vi "Parse Data DualHeading(SubVI).vi"(11 "Parse Data Array":string[](array[string])) -> (3 "Heading":dbl)   [LabVIEW 2019]
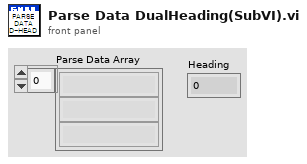
[diagram p1: front panel]
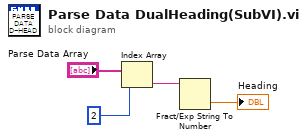
[diagram p0: block diagram]
diagram:
  n1 = Index Array(array="Parse Data Array", index=2) -> (element=w2:string)
  n2 = Fract/Exp String To Number(string=w2) -> (number=→"Heading":dbl)  [unwired: 4 out]
